vi "Vision Research Phantom Series Delay n mSec.vi"(1 "Milliseconds to Wait (0)":u32, 11 "Error In (no error)":errorcluster) -> (15 "Error Out":errorcluster)   [LabVIEW 2013, in "VRI.lvlib"]
doc: "This VI will force a delay of the specified number of milliseconds. Use the error cluster for data flow in the calling VI.\n\nWritten by:\nBLOOMY CONTROLS, INC\nWINDSOR, CT 06095, USA\n860-298-9925\nwww.bloomy.com\nV1.0.0\nMay, 2004"
uses:
  VRI.lvlib
panel:
  # "For instructions on the use of this VI, press Ctrl+H to display the help window and move the mouse over the icon, controls, and indicators"
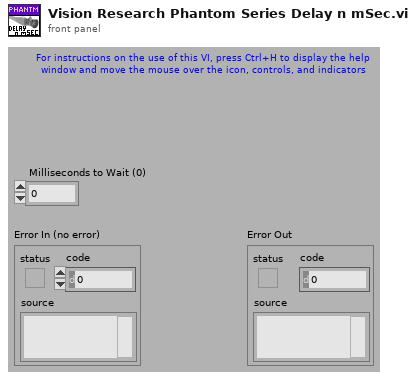
[diagram p1: front panel]
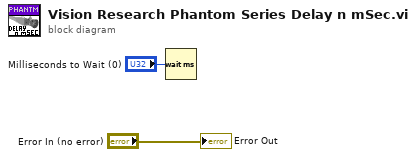
[diagram p0: block diagram]
diagram:
  n1 = Wait (ms)(milliseconds to wait="Milliseconds to Wait (0)") -> ()  [unwired: 1 out]
  "Error Out" <- "Error In (no error)"
